vi "globalTearDown.vi"(8 "error in (no error)":errorcluster, 11 "Create Execution Unit in":refnum<class "Create Execution Unit.lvclass">) -> (0 "error out":errorcluster, 3 "Create Execution Unit out":refnum<class "Create Execution Unit.lvclass">)   [LabVIEW 2020, in "Create Execution Unit.lvclass"]
uses:
  Create Execution Unit.lvclass
  Hardware API/Global - Disable Hardware API Constant.vi
  Hardware API/AIM MIL-STD-1553 Hardware API.lvlib
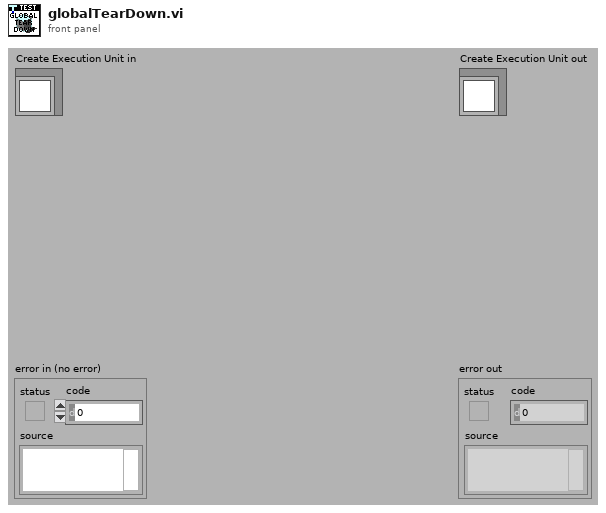
[diagram p1: front panel]
types:
  T1 = enum16{"Enabled (Default)", "Disabled for Unit Testing"}
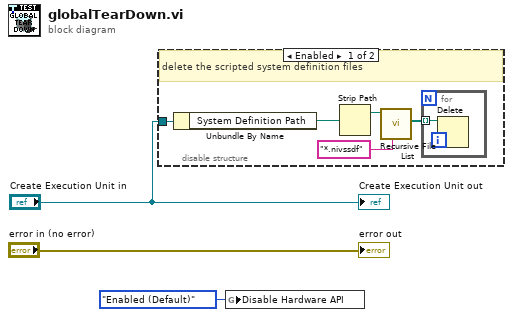
[diagram p0: block diagram]
diagram:
  n1 = disable-structure shown="Enabled" {
    disable-tunnel: "Create Execution Unit in" -> [w8 _]
    frame Enabled {
      # "delete the scripted system definition files"
      n2 = Unbundle By Name(w8) -> ("System Definition Path"=w5:path)
      n3 = Strip Path(path=w5) -> (stripped path=w4:path)  [unwired: 1 out]
      n4 = call <vilib>:"Recursive File List.vi"("pattern"="*.nivssdf", "Folder Path"=w4) -> ("All Files in Dir"=w6:path[])  [unwired: 5 in, 4 out]
      n5 = for {
        tunnel: w6 -> [w9] mode=indexing
        n6 = Delete(path (use dialog)=w9) -> ()  [unwired: 4 in, 3 out]
      }
    }
    frame Disabled {
    }
  }
  n7 = global write "Global - Disable Hardware API Constant.vi" "Disable Hardware API"(T1."Enabled (Default)" ("Disable Hardware API")) -> ()
  "error out" <- "error in (no error)"
  "Create Execution Unit out" <- "Create Execution Unit in"
